vi "blink1.vi"() -> ()   [LabVIEW 2013]
panel:
  in  "OK Button 10":bool
  in  "OK Button 9":bool
  in  "OK Button 8":bool
  in  "OK Button 7":bool
  in  "OK Button 6":bool
  in  "OK Button 5":bool
  in  "OK Button 4":bool
  in  "OK Button 3":bool
  in  "OK Button 2":bool
  in  "OK Button":bool
  in  "stop":bool
  out "Boolean":bool
  # "Page 2"
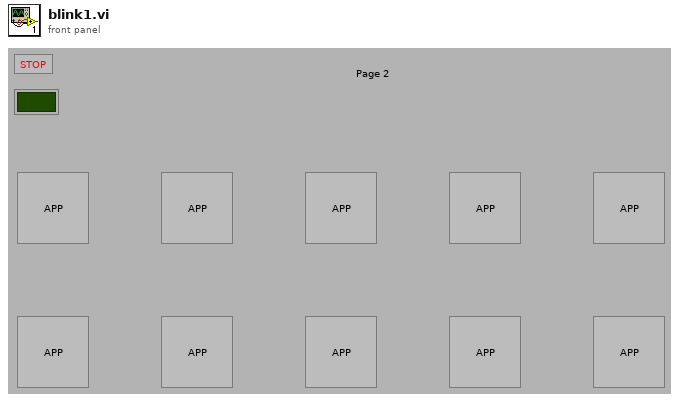
[diagram p1: front panel]
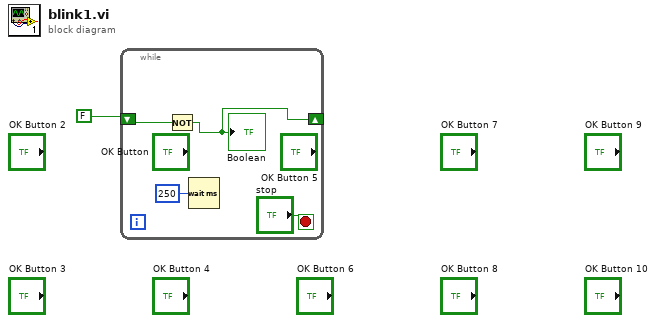
[diagram p0: block diagram]
diagram:
  n1 = while {
    shift-right: [w3] -> _
    shift-left: FALSE ("Boolean") -> [w4]
    stop <- "stop" stop-if-true
    n2 = Not(x=w4) -> (.not. x?=w3:bool)
    "Boolean" <- w3
    n3 = Wait (ms)(milliseconds to wait=u32 250) -> ()  [unwired: 1 out]
  }
